vi "WinHWND.vi"() -> ()   [LabVIEW 2023]
doc: "This function flashes the example VI's title bar 5 times. The HWND for the example VI is returned in output.\n\nFor information on the data types used for the DLL function, right-click on the Call Library Function node and choose Configure."
uses:
  CLF_Example.dll
panel:
  out "output":u64
  # "See the block diagram for more information."
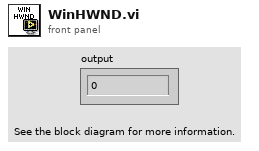
[diagram p1: front panel]
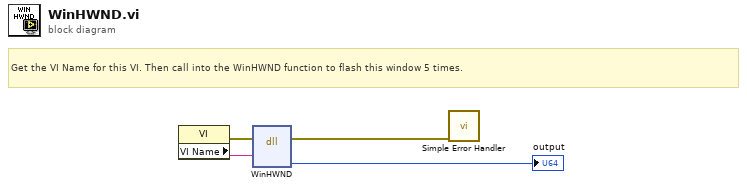
[diagram p0: block diagram]
diagram:
  # "Get the VI Name for this VI. Then call into the WinHWND function to flash this window 5 times."
  n1 = property class="VI"() -> (error out=w2:errorcluster, "VI Name"=w4:string)  [unwired: 2 in, 1 out]
  n2 = dll-call lib="c:/dev/_r/4/eng/lv-core/lvpostprocessingd/lv_mc_x86_64/dist_i386/examples/Connectivity/Libraries and Executables/DLL Calling VIs/CLF_Example**.*" fn="WinHWND"(error in=w2, "name"=w4) -> (error out=w1:errorcluster, "output"=→"output":u64)  [unwired: 3 in, 3 out]
  n3 = call <vilib>:"Simple Error Handler.vi"("error in (no error)"=w1) -> ()  [unwired: 4 in, 5 out]
